vi "ANALOGICO.vi"(9 "ANALOGICO":T1={"ANALOGICO CANALES"=[], "Numero de muestras"=1000, "Frecuencia de muestreo"=1000}, 11 "Adquisicion tiempo":i32) -> ()   [LabVIEW 2020, in "Settings.lvlib"]
uses:
  Settings.lvlib
  Acquisition/cluster analogico.ctl
  <vilib>/drjdpowell/SQLite Library/SQL Connection/Open (path).vi
  <vilib>/drjdpowell/SQLite Library/SQL Connection/Open (string).vi
  <vilib>/AdvancedString/Path To Command Line String.vi
  <vilib>/drjdpowell/SQLite Library/SQL Connection/Execute SQL (No results).vi
  <vilib>/drjdpowell/SQLite Library/SQL Connection/Connection.lvclass
  <vilib>/drjdpowell/SQLite Library/SQLite.lvlib
  Acquisition/CONTROLS.lvlib
panel:
  out "error out":errorcluster
  in  "error in (no error)":errorcluster
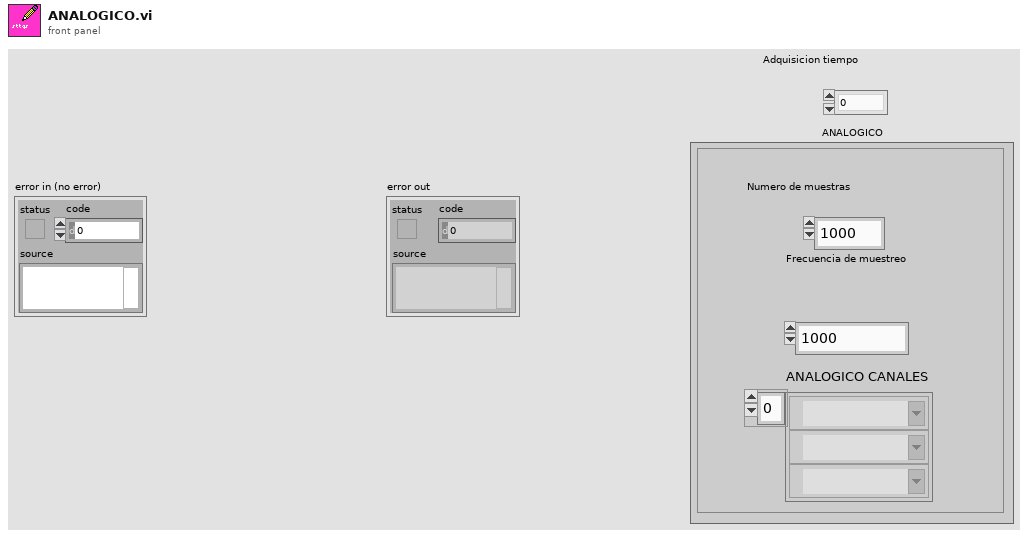
[diagram p1: front panel]
types:
  T1 = typedef "Acquisition.lvlib/CONTROLS.lvlib/cluster analogico.ctl" = cluster{"ANALOGICO CANALES":tag[], "Numero de muestras":u32, "Frecuencia de muestreo":u32}
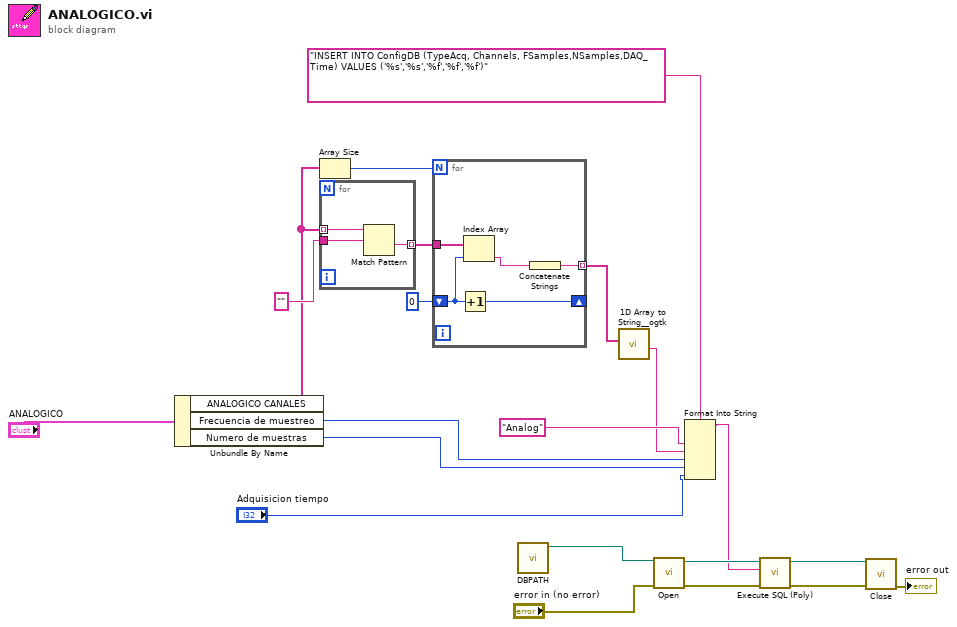
[diagram p0: block diagram]
diagram:
  n1 = Unbundle By Name("ANALOGICO") -> ("ANALOGICO CANALES"=w8:tag[], "Frecuencia de muestreo"=w7:u32, "Numero de muestras"=w6:u32)
  n2 = Array Size(array=w8) -> (size(s)=w12:i32)
  n3 = for {
    tunnel: w8 -> [w24] mode=indexing
    tunnel: [w23] -> w11 mode=indexing
    tunnel: "" ("regular expression") -> [w22]
    n4 = Match Pattern(string=w24, regular expression=w22) -> (after substring=w23:string)  [unwired: 1 in, 3 out]
  }
  n5 = for {
    N: w12 -> [_]
    shift-right: [w27] -> _
    shift-left: 0 -> [w28]
    tunnel: w11 -> [w29]
    tunnel: [w25] -> w13 mode=indexing
    n6 = Increment(x=w28) -> (x+1=w27:i32)
    n7 = Index Array(array=w29, index=w28) -> (element=w26:string)
    n8 = Concatenate Strings(w26) -> (w25:string)
  }
  n9 = call "DBPATH.vi"() -> ("appended path"=w3:path)  [unwired: 11 in]
  n10 = call <userlib>:"1D Array to String__ogtk.vi"("Array of Strings"=w13) -> ("delimited string"=w4:string)  [unwired: 10 in]
  n11 = call-poly <vilib>:"Open.vi"("error in (no error)"="error in (no error)", "db file"=w3) -> ("error out"=w21:errorcluster, "SQLite Connection"=w19:refnum<class "Connection.lvclass">)  [unwired: 8 in]
  n12 = Format Into String(format string="INSERT INTO ConfigDB (TypeAcq, Channels, FSamples,NSamples,DAQ_Time) VALUES ('%s','%s','%f','%f','%f')", "Analog" ("input 1"), w4, w7, w6, "Adquisicion tiempo") -> (resulting string=w15:string)  [unwired: 2 in, 1 out]
  n13 = call-poly <vilib>:"Execute SQL (Poly).vi"("error in (no error)"=w21, "SQL"=w15, "SQLite Connection in"=w19) -> ("error out"=w20:errorcluster, "SQLite Connection"=w18:refnum<class "Connection.lvclass">)  [unwired: 7 in]
  n14 = call-dynamic "Close.vi"("error in (no error)"=w20, "SQLite Connection in"=w18) -> ("error out"=→"error out":errorcluster)  [unwired: 9 in]
